vi "Create graphs.vi"(0 "Acquired Data":T1) -> (14 "Iin ripples":waveform(dbl)[](array[waveform]), 15 "Iout ripples":waveform(dbl)[](array[waveform]), 16 "Iouts 60Hz":waveform(dbl)[](array[waveform]), 17 "Phase 1 60 Hz V and I":waveform(dbl)[](array[waveform]), 18 "Phase 2 60 Hz V and I":waveform(dbl)[](array[waveform]), 19 "Phase 3 60 Hz V and I":waveform(dbl)[](array[waveform]))   [LabVIEW 2019, in "Main.lvclass"]
doc: "Developed by Kevin Thompson\nkevin@thompsonengineering.net\n\nCopyright 2020\nThompson Engineering, LLC"
uses:
  Main.lvclass
  DataTypes/raw data variables.ctl
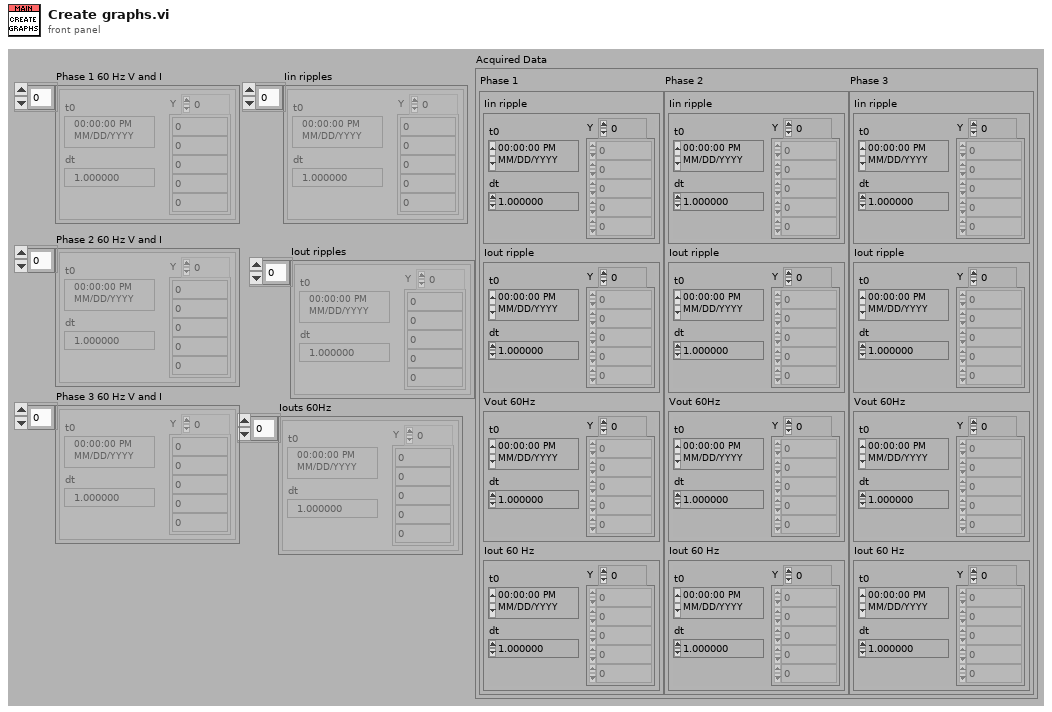
[diagram p1: front panel]
types:
  T1 = typedef "Main.lvclass/raw data variables.ctl" = cluster{"Phase 1":cluster{"Iin ripple":waveform(dbl), "Iout ripple":waveform(dbl), "Vout 60Hz":waveform(dbl), "Iout 60 Hz":waveform(dbl)}, "Phase 2":cluster{"Iin ripple":waveform(dbl), "Iout ripple":waveform(dbl), "Vout 60Hz":waveform(dbl), "Iout 60 Hz":waveform(dbl)}, "Phase 3":cluster{"Iin ripple":waveform(dbl), "Iout ripple":waveform(dbl), "Vout 60Hz":waveform(dbl), "Iout 60 Hz":waveform(dbl)}}
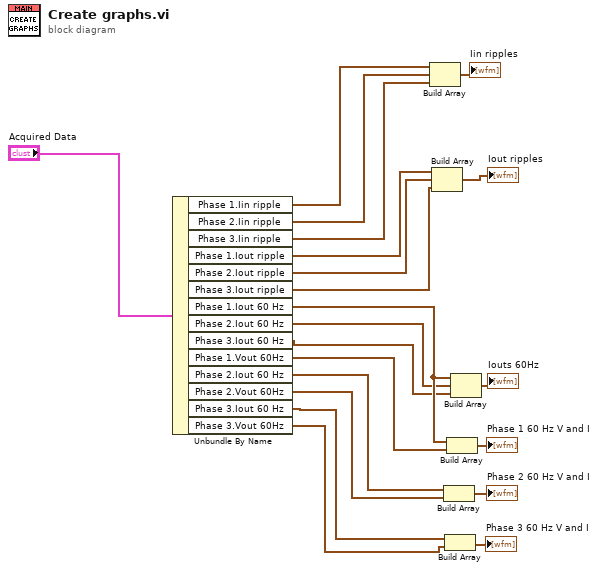
[diagram p0: block diagram]
diagram:
  n1 = Unbundle By Name("Acquired Data") -> ("Phase 1.Iin ripple"=w20:waveform(dbl), "Phase 2.Iin ripple"=w19:waveform(dbl), "Phase 3.Iin ripple"=w10:waveform(dbl), "Phase 1.Iout ripple"=w16:waveform(dbl), "Phase 2.Iout ripple"=w17:waveform(dbl), "Phase 3.Iout ripple"=w9:waveform(dbl), "Phase 1.Iout 60 Hz"=w13:waveform(dbl), "Phase 2.Iout 60 Hz"=w12:waveform(dbl), "Phase 3.Iout 60 Hz"=w8:waveform(dbl), "Phase 1.Vout 60Hz"=w7:waveform(dbl), "Phase 2.Iout 60 Hz"=w6:waveform(dbl), "Phase 2.Vout 60Hz"=w5:waveform(dbl), "Phase 3.Iout 60 Hz"=w3:waveform(dbl), "Phase 3.Vout 60Hz"=w2:waveform(dbl))
  n2 = Build Array(w20, w19, w10) -> (→"Iin ripples":waveform(dbl)[])
  n3 = Build Array(w16, w17, w9) -> (→"Iout ripples":waveform(dbl)[])
  n4 = Build Array(w6, w5) -> (→"Phase 2 60 Hz V and I":waveform(dbl)[])
  n5 = Build Array(w3, w2) -> (→"Phase 3 60 Hz V and I":waveform(dbl)[])
  n6 = Build Array(w13, w7) -> (→"Phase 1 60 Hz V and I":waveform(dbl)[])
  n7 = Build Array(w13, w12, w8) -> (→"Iouts 60Hz":waveform(dbl)[])
